vi "OB Read.vi"(7 "ReadDataLen":u32, 9 "pReadData":T1, 10 "Channel":u8, 11 "DevHandle":i32) -> (1 "pReadData out":T1, 3 "function return":i32)   [LabVIEW 2010, in "usb2openbus.lvlib"]
doc: "int WINAPI OB_Read(int DevHandle, unsigned char Channel,OB_DATA *pReadData,unsigned int ReadDataLen);"
uses:
  usb2openbus.lvlib
  USB2XXX.dll
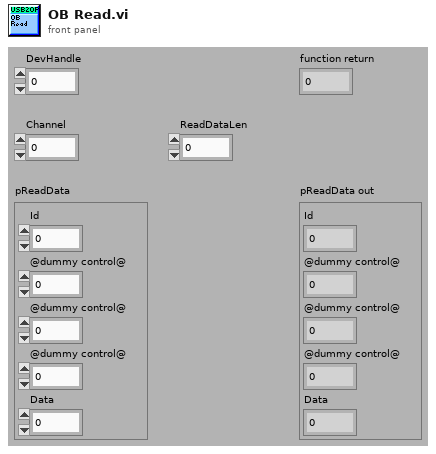
[diagram p1: front panel]
types:
  T1 = cluster{"Id":i8, "@dummy control@":i8, "@dummy control@":i8, "@dummy control@":i8, "Data":u32}
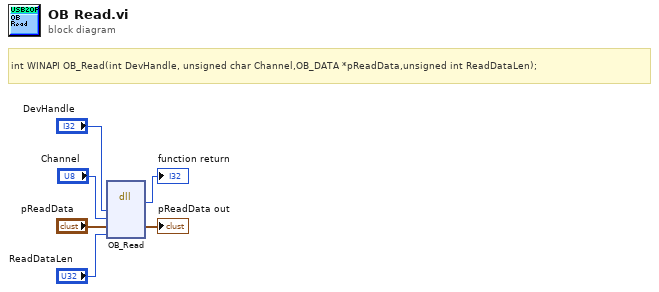
[diagram p0: block diagram]
diagram:
  # "int WINAPI OB_Read(int DevHandle, unsigned char Channel,OB_DATA *pReadData,unsigned int ReadDataLen);"
  n1 = dll-call lib="F:/OtherWork/STM32/USB2XXX_Example/trunk/Labview/PublicFiles/usb2openbus/USB2XXX.*" fn="OB_Read"("DevHandle"="DevHandle", "Channel"="Channel", "pReadData"="pReadData", "ReadDataLen"="ReadDataLen") -> (→"function return":i32, "pReadData"=→"pReadData out":T1)  [unwired: 6 in, 2 out]
